vi "mro apply Command.vi"(8 "error in (no error)":errorcluster, 10 "trig":i8) -> (0 "error out":errorcluster, 1 "status out":i32, 2 "function return":i8)   [LabVIEW 2016, in "mirao52e_32bit.lvlib"]
doc: "MIRAOEXPORT MroBoolean MIRAOCALL mro_applyCommand( \n MroCommand command, \n MroBoolean trig,\n int* status\n );"
uses:
  mirao52e_32bit.lvlib
  MRO Error codes.ctl
  mirao52e.dll
panel:
  out "Command array":dbl[](array[numeric])
  out "MRO Error code":T1
  out "MRO_TRUE ?":bool
  # "Apply Command"
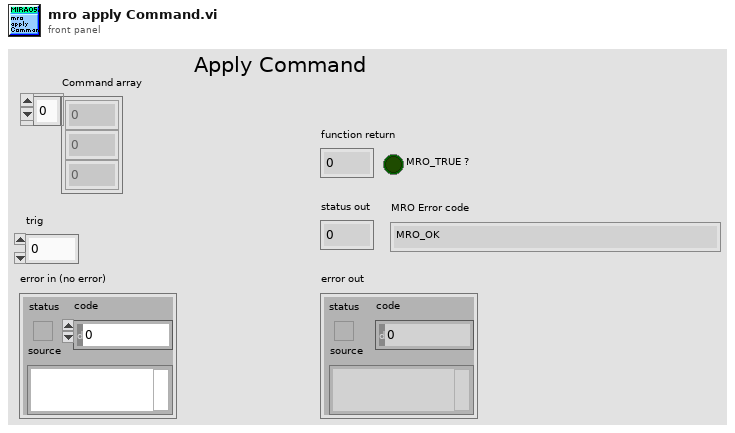
[diagram p1: front panel]
types:
  T1 = typedef "MRO Error codes.ctl" = enum16{"MRO_OK", "MRO_UNKNOWN_ERROR", "MRO_DEVICE_NOT_OPENED_ERROR", "MRO_DEFECTIVE_DEVICE_ERROR", "MRO_DEVICE_ALREADY_OPENED_ERROR", "MRO_DEVICE_IO_ERROR", "MRO_DEVICE_LOCKED_ERROR", "MRO_DEVICE_DISCONNECTED_ERROR", "MRO_DEVICE_DRIVER_ERROR", "MRO_FILE_EXISTS_ERROR", "MRO_FILE_FORMAT_ERROR", "MRO_FILE_IO_ERROR", "MRO_INVALID_COMMAND_ERROR", "MRO_NULL_POINTER_ERROR", "MRO_OUT_OF_BOUNDS_ERROR", "MRO_OPERATION_ONGOING_ERROR", "MRO_SYSTEM_ERROR", "MRO_UNAVAILABLE_DATA_ERROR", "MRO_UNDEFINED_VALUE_ERROR", "MRO_OUT_OF_SPECIFICATIONS_ERROR", "MRO_FILE_FORMAT_VERSION_ERROR", "MRO_USB_INVALID_HANDLE", "MRO_USB_DEVICE_NOT_FOUND", "MRO_USB_DEVICE_NOT_OPENED", "MRO_USB_IO_ERROR", "MRO_USB_INSUFFICIENT_RESOURCES", "MRO_USB_INVALID_BAUD_RATE", "MRO_USB_NOT_SUPPORTED", "MRO_FILE_IO_EACCES", "MRO_FILE_IO_EAGAIN", "MRO_FILE_IO_EBADF", "MRO_FILE_IO_EINVAL", "MRO_FILE_IO_EMFILE", "MRO_FILE_IO_ENOENT", "MRO_FILE_IO_ENOMEM", "MRO_FILE_IO_ENOSPC"}
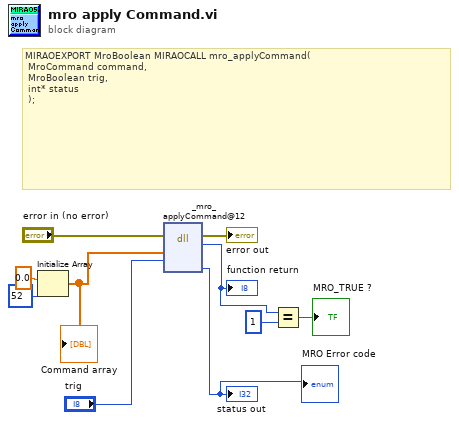
[diagram p0: block diagram]
diagram:
  # "MIRAOEXPORT MroBoolean MIRAOCALL mro_applyCommand( \n\tMroCommand command, \n\tMroBoolean trig,\n\tint* status\n\t);"
  n1 = Initialize Array(0.0 ("element"), 52 ("dimension size")) -> (w6:dbl[])
  "Command array" <- w6
  n2 = dll-call lib="C:/Users/nvladim/Documents/Nikita-MDC/code/LabView/miraoDriver_32bit/mirao52e.*" fn="_mro_applyCommand@12"(error in="error in (no error)", "command"=w6, "trig"="trig") -> (error out=→"error out":errorcluster, "return type"=w2:i8, "status"=→"status out" →"MRO Error code":i32)  [unwired: 5 in, 1 out]
  "function return" <- w2
  n3 = Equal?(x=w2, y=i8 1) -> (x = y?=→"MRO_TRUE ?":bool)
